vi "TCP通讯.vi"(7 "service name":string caption="服务名称", 8 "error in":errorcluster caption="错误输入（无错误）", 9 "数据输入":string, 10 "选项":enum16{"NA", "侦听", "读取", "写入", "关闭"}(ring)=enum."侦听", 11 "connection ID in":refnum<k5>) -> (0 "error out":errorcluster caption="错误输出", 1 "数据输出":string, 2 "send ok":bool, 3 "connection ID out":refnum<k5>, 4 "open com":bool)   [LabVIEW 2017]
panel:
  out "写入的字节":i32
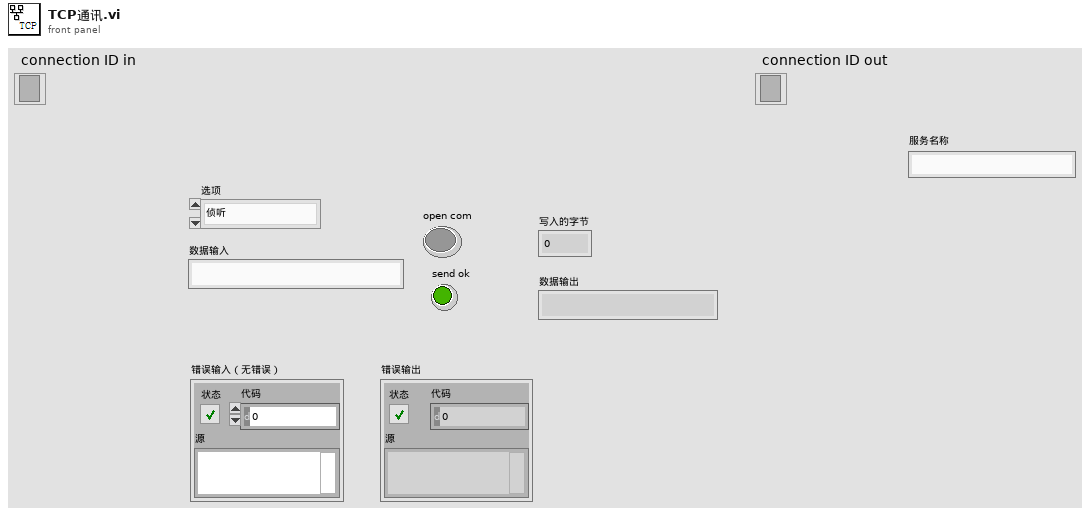
[diagram p1: front panel]
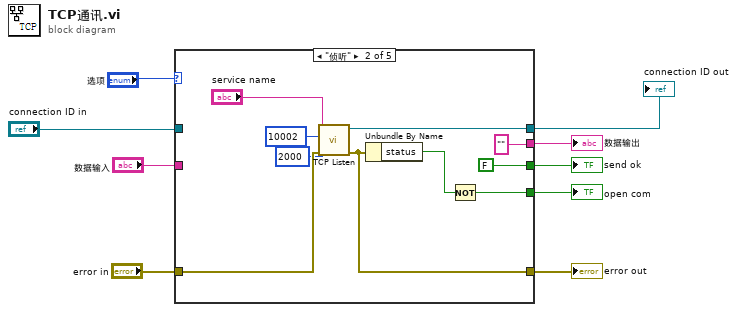
[diagram p0: block diagram]
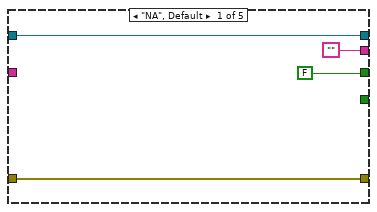
[diagram p2: hidden frame]
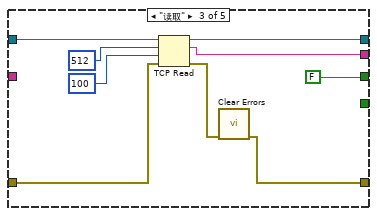
[diagram p3: hidden frame]
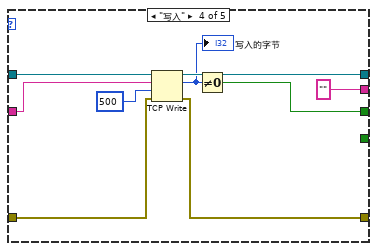
[diagram p4: hidden frame]
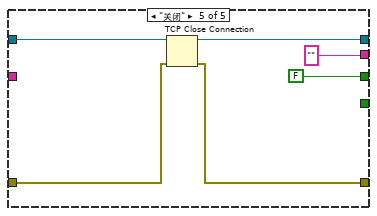
[diagram p5: hidden frame]
diagram:
  n1 = case shown="\"侦听\"" "选项" {
    tunnel: [w13 w21 w29 w39 w46] -> w2
    tunnel: "connection ID in" -> [w13 _ w30 w40 w47]
    tunnel: "error in" -> [w11 w18 w28 w38 w45]
    tunnel: [w11 w17 w25 w33 w44] -> w7
    tunnel: ["" "" w24 "" ""] -> w4
    tunnel: "数据输入" -> [_ _ _ w34 _]
    tunnel: [FALSE FALSE FALSE w37 FALSE] -> w5
    tunnel: [_ w16 _ _ _] -> w3
    frame "NA", Default {
    }
    frame "侦听" {
      n2 = call <vilib>:"TCP Listen.vi"("error in (no error)"=w18, "timeout ms (wait forever: -1)"=2000, "port"=u16 10002, "service name"="service name") -> ("error out"=w17:errorcluster, "connection ID"=w21:refnum<k5>)  [unwired: 3 in, 3 out]
      n3 = Unbundle By Name(w17) -> ("status"=w22:bool)
      n4 = Not(x=w22) -> (.not. x?=w16:bool)
    }
    frame "读取" {
      n5 = TCP Read(connection ID=w30, bytes to read=512 ("读取的字节"), error in (no error)=w28, 9:100 ("超时毫秒(25000)")) -> (connection ID out=w29:refnum<k5>, data out=w24:string, error out=w26:errorcluster)  [unwired: 1 in]
      n6 = call <vilib>:"Clear Errors.vi"("error in (no error)"=w26) -> ("error out"=w25:errorcluster)  [unwired: 5 in, 1 out]
    }
    frame "写入" {
      n7 = TCP Write(connection ID=w40, data in=w34, error in (no error)=w38, 9:500 ("超时毫秒(25000)")) -> (connection ID out=w39:refnum<k5>, bytes written=w35:i32, error out=w33:errorcluster)
      "写入的字节" <- w35
      n8 = Not Equal To 0?(x=w35) -> (x != 0?=w37:bool)
    }
    frame "关闭" {
      n9 = TCP Close Connection(connection ID=w47, error in (no error)=w45) -> (connection ID out=w46:refnum<k5>, error out=w44:errorcluster)  [unwired: 1 in]
    }
  }
  "数据输出" <- w4
  "error out" <- w7
  "send ok" <- w5
  "open com" <- w3
  "connection ID out" <- w2
